vi "AddToQueue.vi"(0 "Cmd":string, 3 "ROS":T1, 4 "Type":enum16{"topic", "node", "ToFIFO"}(ring)) -> (5 "ROS out":T1)   [LabVIEW 2012]
uses:
  <userlib>/ROS for LabVIEW Software/ROS/Code/SubVIs/_ROSControl.ctl
  <userlib>/ROS for LabVIEW Software/ROS/Code/SubVIs/_ROSDirection.ctl
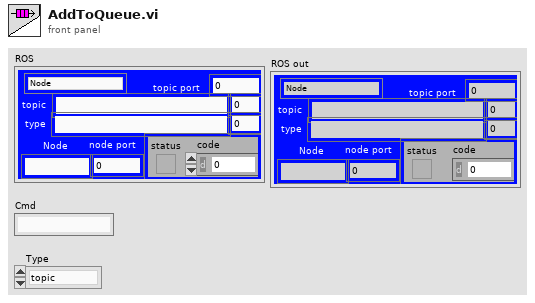
[diagram p1: front panel]
types:
  T1 = typedef "_ROSControl.ctl" = cluster{"topic port":u16, "Node":string, "topic":string, "type":string, "node port":u16, "error ":errorcluster, "Direction":T2, "Update (ms)":u16, "FIFO size":u16}
  T2 = typedef "_ROSDirection.ctl" = enum16{"Node", "Publisher", "Subscriber", "ServiceClient", "ServiceProvider"}
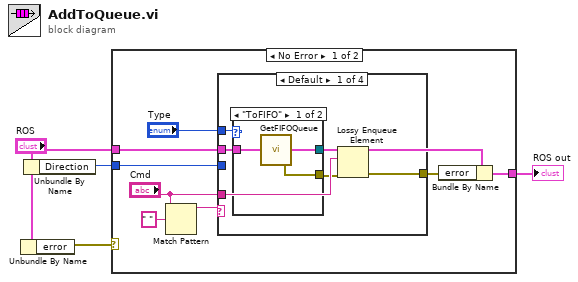
[diagram p0: block diagram]
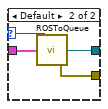
[diagram p2: hidden frame]
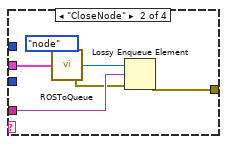
[diagram p3: hidden frame]
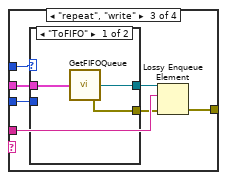
[diagram p4: hidden frame]
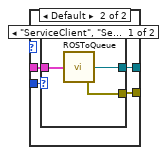
[diagram p5: hidden frame]
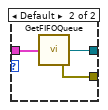
[diagram p6: hidden frame]
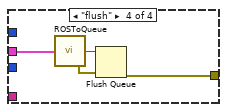
[diagram p7: hidden frame]
diagram:
  n1 = Unbundle By Name("ROS") -> ("error"=w3:errorcluster)
  n2 = Unbundle By Name("ROS") -> ("Direction"=w1:T2)
  n3 = case shown="No Error" w3 {
    tunnel: "ROS" -> [w9 w56]
    tunnel: [w7 w56] -> w4
    tunnel: w1 -> [w5 _]
    frame No Error {
      n4 = Match Pattern(string="Cmd", regular expression=" ") -> (before substring=w10:string)  [unwired: 1 in, 3 out]
      n5 = case shown="Default" w10 {
        tunnel: "Cmd" -> [w18 w31 w38 _]
        tunnel: [w14 w27 w34 w53] -> w8
        tunnel: w9 -> [w17 w29 w36 w55]
        tunnel: "Type" -> [w15 _ w33 _]
        tunnel: w5 -> [_ _ w35 _]
        frame Default {
          n6 = case shown="\"ToFIFO\"" w15 {
            selector: w15 -> [_ w23]
            tunnel: w17 -> [w21 w25]
            tunnel: [w20 w24] -> w16
            tunnel: [w19 w22] -> w13
            frame "ToFIFO" {
              n7 = call <userlib>:"GetFIFOQueue.vi"("ROS"=w21) -> ("error out"=w19:errorcluster, "queue out"=w20:refnum<queue>)  [unwired: 3 in]
            }
            frame Default {
              n8 = call <userlib>:"ROSToQueue.vi"("ROS"=w25, "Name"=w23) -> ("error out"=w22:errorcluster, "queue"=w24:refnum<queue>)  [unwired: 2 in]
            }
          }
          n9 = Lossy Enqueue Element(queue=w16, element=w18, error in (no error)=w13) -> (error out=w14:errorcluster)  [unwired: 3 out]
        }
        frame "CloseNode" {
          n10 = call <userlib>:"ROSToQueue.vi"("ROS"=w29, "Name"=enum16{"topic", "node"}."node" ("Type 2")) -> ("error out"=w26:errorcluster, "queue"=w28:refnum<queue>)  [unwired: 2 in]
          n11 = Lossy Enqueue Element(queue=w28, element=w31, error in (no error)=w26) -> (error out=w27:errorcluster)  [unwired: 3 out]
        }
        frame "repeat", "write" {
          n12 = case shown="\"ToFIFO\"" w33 {
            tunnel: [w40 w45] -> w37
            tunnel: w36 -> [w41 w44]
            tunnel: w35 -> [_ w43]
            tunnel: [w39 w42] -> w32
            frame "ToFIFO" {
              n13 = call <userlib>:"GetFIFOQueue.vi"("ROS"=w41) -> ("error out"=w39:errorcluster, "queue out"=w40:refnum<queue>)  [unwired: 3 in]
            }
            frame Default {
              n14 = case shown="\"ServiceClient\", \"ServiceProvider\"" w43 {
                tunnel: [w47 w51] -> w45
                tunnel: w44 -> [w48 w50]
                tunnel: [w46 w49] -> w42
                frame "ServiceClient", "ServiceProvider" {
                  n15 = call <userlib>:"ROSToQueue.vi"("ROS"=w48) -> ("error out"=w46:errorcluster, "queue"=w47:refnum<queue>)  [unwired: 3 in]
                }
                frame Default {
                  n16 = call <userlib>:"GetFIFOQueue.vi"("ROS"=w50) -> ("error out"=w49:errorcluster, "queue out"=w51:refnum<queue>)  [unwired: 3 in]
                }
              }
            }
          }
          n17 = Lossy Enqueue Element(queue=w37, element=w38, error in (no error)=w32) -> (error out=w34:errorcluster)  [unwired: 3 out]
        }
        frame "flush" {
          n18 = call <userlib>:"ROSToQueue.vi"("ROS"=w55) -> ("error out"=w52:errorcluster, "queue"=w54:refnum<queue>)  [unwired: 3 in]
          n19 = Flush Queue(queue=w54, error in (no error)=w52) -> (error out=w53:errorcluster)  [unwired: 2 out]
        }
      }
      n20 = Bundle By Name(cluster=w9, "error"=w8) -> (w7:T1)
    }
    frame Error {
    }
  }
  "ROS out" <- w4
